vi "AcurrDataIn.vi"(7 "通道":u16(ring) items=["CH1", "CH2", "CH3", "CH4", "CH5", "CH6", "CH7", "CH8", "CH9", "CH10"], 8 "error in (no error)":errorcluster, 9 "温度":dbl, 10 "测试类型":string, 11 "数组":dbl[](array[numeric])) -> (0 "error out":errorcluster, 3 "记录时间":string)   [LabVIEW 2014]
uses:
  <vilib>/addons/database/Connection.llb/DB Tools Open Connec (String).vi
  <vilib>/addons/database/Connection.llb/Conn Execute.vi
  <vilib>/addons/database/Recordset.llb/Rec Destroy - Connection.vi
  <vilib>/addons/database/NI_Database_API.lvlib
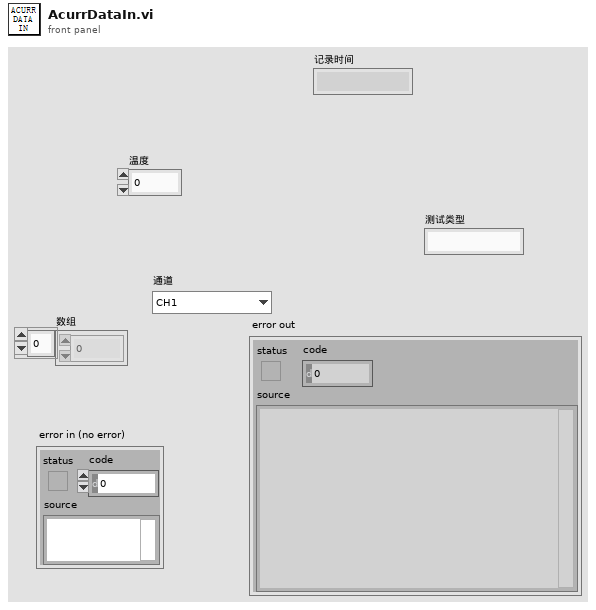
[diagram p1: front panel]
types:
  T1 = typedef "NI_Database_API.lvlib/Conn ObjectReference.ctl" = refnum<k1>
  T2 = typedef "NI_Database_API.lvlib/Rec ObjectReference.ctl" = refnum<k1>
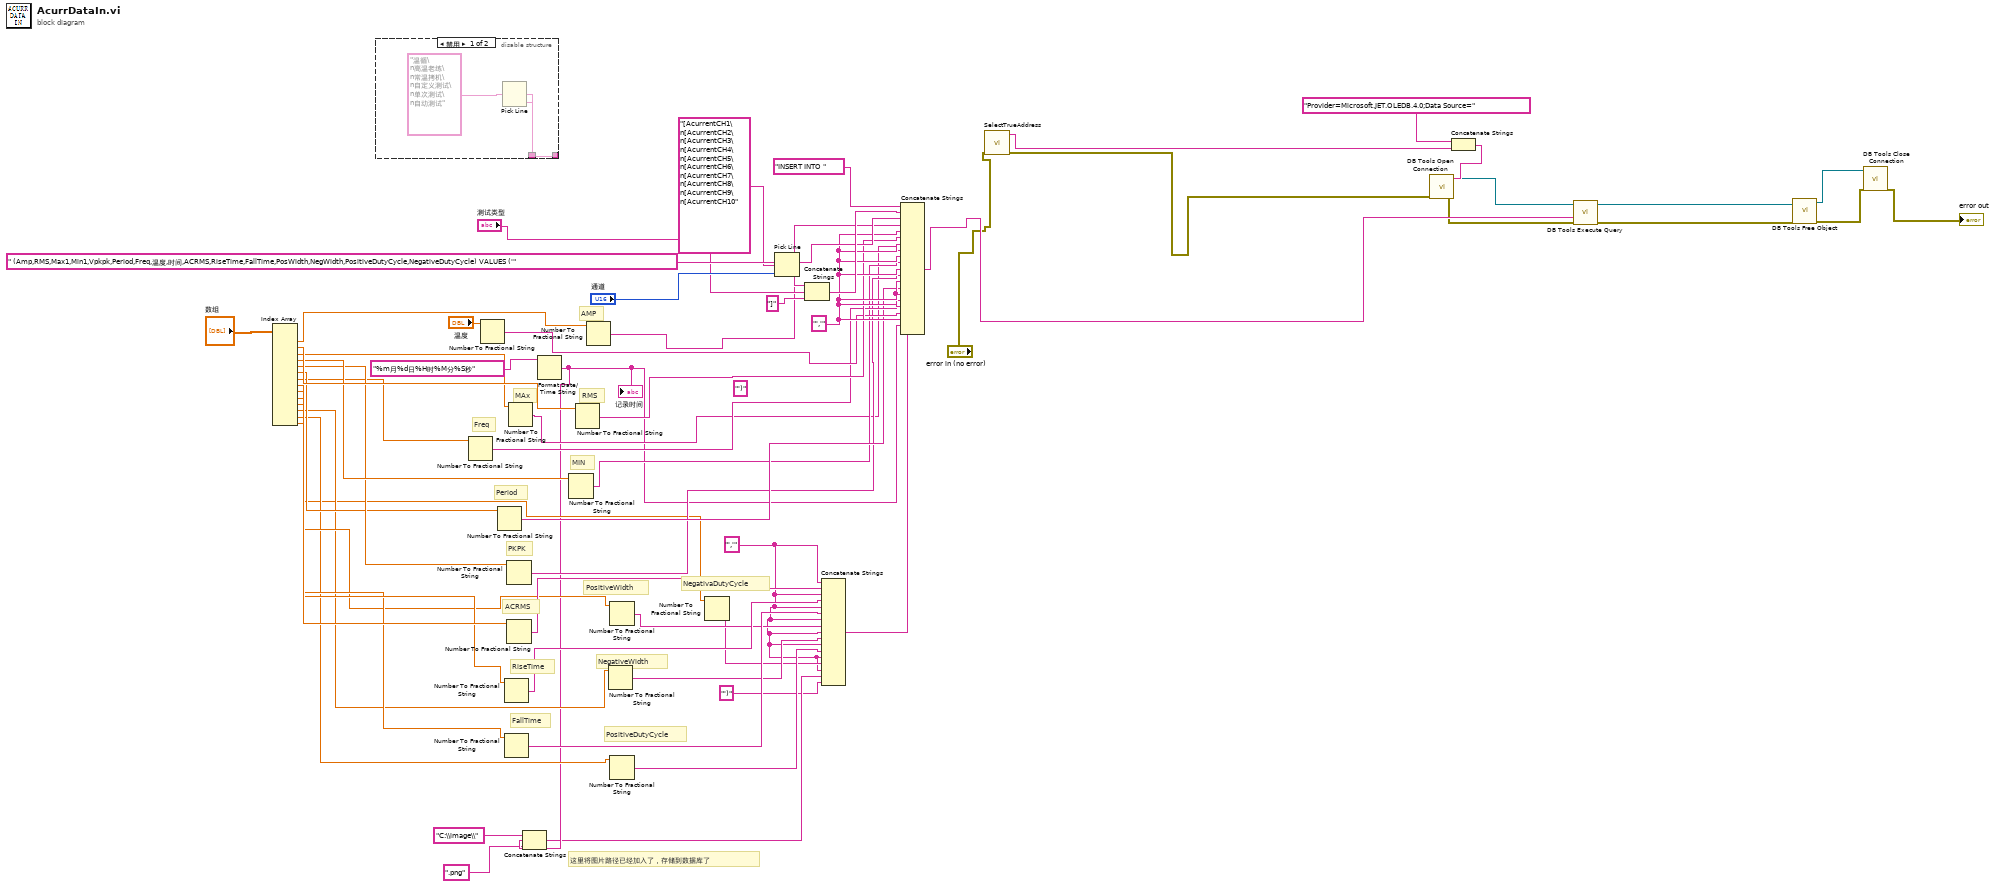
[diagram p0: block diagram]
diagram:
  w3 = "','"
  w54 = "','"
  (unwired) "')"
  # "这里将图片路径已经加入了，存储到数据库了"
  # "NegativaDutyCycle"
  # "PositiveDutyCycle"
  # "NegativeWidth"
  # "PositiveWidth"
  # "FallTime"
  # "RiseTime"
  # "ACRMS"
  # "Freq"
  # "Period"
  # "PKPK"
  # "MIN"
  # "MAx"
  # "RMS"
  # "AMP"
  n1 = Index Array(array="数组") -> (element #1=w20:dbl, element #2=w19:dbl, element #3=w18:dbl, element #4=w17:dbl, element #5=w16:dbl, element #6=w15:dbl, element #7=w14:dbl, element #8=w13:dbl, element #9=w12:dbl, element #10=w11:dbl, element #11=w10:dbl, element #12=w9:dbl, element #13=w8:dbl, element #14=w7:dbl)  [unwired: 14 in]
  n2 = disable-structure shown="禁用" {
    disable-tunnel: [w64 _] -> _
    disable-tunnel: _ -> [w63 _]
    frame Disabled {
      n3 = Pick Line(multi-line string="温循\n高温老练\n常温拷机\n自定义测试\n单次测试\n自动测试" ("多行字符串"), line index=w63) -> (output string=w64:string)  [unwired: 1 in]
    }
    frame Enabled {
    }
  }
  n4 = Number To Fractional String(number=w14) -> (F-format string=w47:string)  [unwired: 3 in]
  n5 = Number To Fractional String(number="温度") -> (F-format string=w48:string)  [unwired: 3 in]
  n6 = Number To Fractional String(number=w15) -> (F-format string=w46:string)  [unwired: 3 in]
  n7 = Number To Fractional String(number=w12) -> (F-format string=w28:string)  [unwired: 3 in]
  n8 = Number To Fractional String(number=w11) -> (F-format string=w27:string)  [unwired: 3 in]
  n9 = Number To Fractional String(number=w16) -> (F-format string=w45:string)  [unwired: 3 in]
  n10 = Number To Fractional String(number=w13) -> (F-format string=w29:string)  [unwired: 3 in]
  n11 = Number To Fractional String(number=w18) -> (F-format string=w43:string)  [unwired: 3 in]
  n12 = Format Date/Time String(time format string (%c)="%m月%d日%H时%M分%S秒" ("时间格式字符串(%c)")) -> (date/time string=w5:string)  [unwired: 2 in]
  "记录时间" <- w5
  n13 = Concatenate Strings("C:\\image\\", w5, ".png") -> (w2:string)
  n14 = Number To Fractional String(number=w17) -> (F-format string=w44:string)  [unwired: 3 in]
  n15 = Number To Fractional String(number=w19) -> (F-format string=w50:string)  [unwired: 3 in]
  n16 = Number To Fractional String(number=w20) -> (F-format string=w51:string)  [unwired: 3 in]
  n17 = Number To Fractional String(number=w9) -> (F-format string=w25:string)  [unwired: 3 in]
  n18 = Number To Fractional String(number=w10) -> (F-format string=w26:string)  [unwired: 3 in]
  n19 = Number To Fractional String(number=w8) -> (F-format string=w24:string)  [unwired: 3 in]
  n20 = Number To Fractional String(number=w7) -> (F-format string=w23:string)  [unwired: 3 in]
  n21 = Pick Line(multi-line string="[AcurrentCH1\n[AcurrentCH2\n[AcurrentCH3\n[AcurrentCH4\n[AcurrentCH5\n[AcurrentCH6\n[AcurrentCH7\n[AcurrentCH8\n[AcurrentCH9\n[AcurrentCH10" ("多行字符串"), line index="通道") -> (output string=w60:string)  [unwired: 1 in]
  n22 = Concatenate Strings(w60, "测试类型", "]") -> (w59:string)
  n23 = Concatenate Strings(w3, w29, w3, w28, w3, w27, w3, w26, w3, w25, w3, w24, w3, w23, w3, w2, "')") -> (w22:string)
  n24 = Concatenate Strings("INSERT INTO ", w59, " (Amp,RMS,Max1,Min1,Vpkpk,Period,Freq,温度,时间,ACRMS,RiseTime,FallTime,PosWidth,NegWidth,PositiveDutyCycle,NegativeDutyCycle) VALUES ('", w51, w54, w50, w54, w43, w54, w44, w54, w45, w54, w46, w54, w47, w54, w48, w54, w5, w22) -> (w41:string)
  n25 = call "SelectTrueAddress.vi"("error in (no error)"="error in (no error)") -> ("error out"=w30:errorcluster, "元素"=w42:string)  [unwired: 9 in]
  n26 = Concatenate Strings("Provider=Microsoft.JET.OLEDB.4.0;Data Source=", w42) -> (w38:string)
  n27 = call-poly <vilib>:"DB Tools Open Connection.vi"("error in (no error)"=w30, "connection information"=w38) -> ("error out"=w36:errorcluster, "connection reference"=w37:T1)  [unwired: 6 in]
  n28 = call-poly <vilib>:"DB Tools Execute Query.vi"("error in (no error)"=w36, "SQL query"=w41, "connection reference"=w37) -> ("error out"=w34:errorcluster, "recordset reference"=w35:T2)  [unwired: 5 in]
  n29 = call-poly <vilib>:"DB Tools Free Object.vi"("error in (no error)"=w34, "recordset reference"=w35) -> ("error out"=w32:errorcluster, "connection reference"=w33:T1)  [unwired: 8 in]
  n30 = call <vilib>:"DB Tools Close Connection.vi"("error in (no error)"=w32, "connection reference"=w33) -> ("error out"=→"error out":errorcluster)  [unwired: 5 in]
